vi "readBaseCommunicatorSettings.vi"(8 "error in (no error)":errorcluster, 11 "Boot in":refnum<class "Boot.lvclass">) -> (0 "error out":errorcluster, 2 "M1M3SALSettings":T1={"Connection"={"IPAddress"="127.0.0.1", "Port"=0, "StartupScript"="source /usr/ts_sal/setup.env && /usr/ts_sal/test/m1m3/cpp/src/SALPipe %d -1"}}, 3 "Boot out":refnum<class "Boot.lvclass">)   [LabVIEW 2016, in "Boot.lvclass"]
uses:
  Boot.lvclass
  DataTypes/Settings/Base/BaseSALSettings.ctl
  Communicator/DataTypes/M1M3SALSettings.ctl
  Boot.lvclass/Boot.ctl
  Settings/Settings/Setting.lvclass
  Communicator/M1M3SupportCommunicator.lvlib
  DataTypes/Settings/M1M3SupportSettings.lvlib
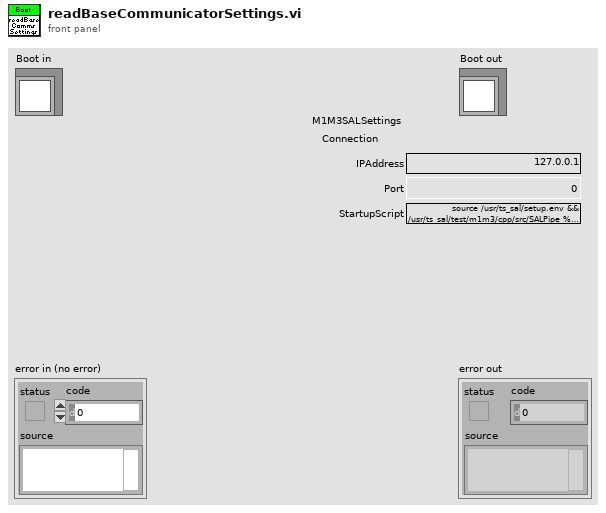
[diagram p1: front panel]
types:
  T1 = typedef "M1M3SupportSettings.lvlib/BaseSALSettings.ctl" = cluster{"Connection":T2}
  T2 = typedef "M1M3SupportCommunicator.lvlib/M1M3SALSettings.ctl" = cluster{"IPAddress":string, "Port":u16, "StartupScript":string}
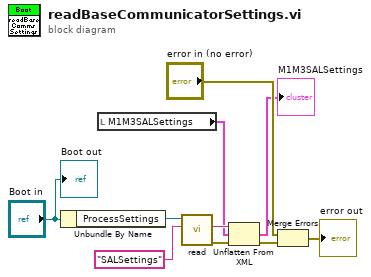
[diagram p0: block diagram]
diagram:
  n1 = Unbundle By Name("Boot in") -> ("ProcessSettings"=w10:refnum<class "Setting.lvclass">)
  n2 = local read "M1M3SALSettings"() -> (w2:T1)
  n3 = call-dynamic "read.vi"("Name"="SALSettings", "BaseSetting in"=w10) -> ("error out"=w6:errorcluster, "XML"=w8:string)  [unwired: 6 in, 2 out]
  n4 = Unflatten From XML(xml string=w8, type=w2, error in (no error)=w6) -> (value=→"M1M3SALSettings":T1, error out=w3:errorcluster)
  n5 = Merge Errors("error in (no error)", w3) -> (→"error out":errorcluster)
  "Boot out" <- "Boot in"
